vi "SSL Detection Ball Coordinate.vi"(11 "Detection Ball":T1) -> (3 "Coordinate":cluster{"x":sgl, "y":sgl, "z":sgl})   [LabVIEW 2016]
uses:
  SSL Detection Ball.ctl
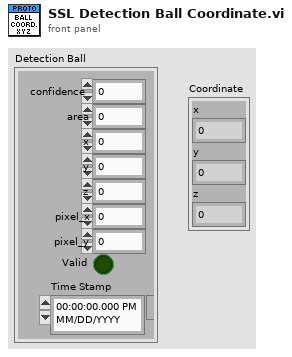
[diagram p1: front panel]
types:
  T1 = typedef "SSL Detection Ball.ctl" = cluster{"x":sgl, "area":u32, "confidence":sgl, "y":sgl, "z":sgl, "pixel_x":sgl, "pixel_y":sgl, "Valid":bool, "Time Stamp":timestamp}
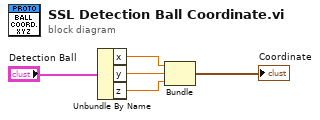
[diagram p0: block diagram]
diagram:
  n1 = Unbundle By Name("Detection Ball") -> ("x"=w2:sgl, "y"=w3:sgl, "z"=w4:sgl)
  n2 = Bundle("x"=w2, "y"=w3, "z"=w4) -> (→"Coordinate":cluster{"x":sgl, "y":sgl, "z":sgl})  [unwired: 1 in]
